vi "Write scan data array.vi"(8 "error in (no error)":errorcluster, 10 "scan data array":T1, 11 "Analysis in":refnum<class "Analysis.lvclass">) -> (0 "error out":errorcluster, 3 "Analysis out":refnum<class "Analysis.lvclass">)   [LabVIEW 2017, in "Analysis.lvclass"]
uses:
  Analysis.lvclass
  ScanDataArray_new.ctl
  Analysis.lvclass/Analysis.ctl
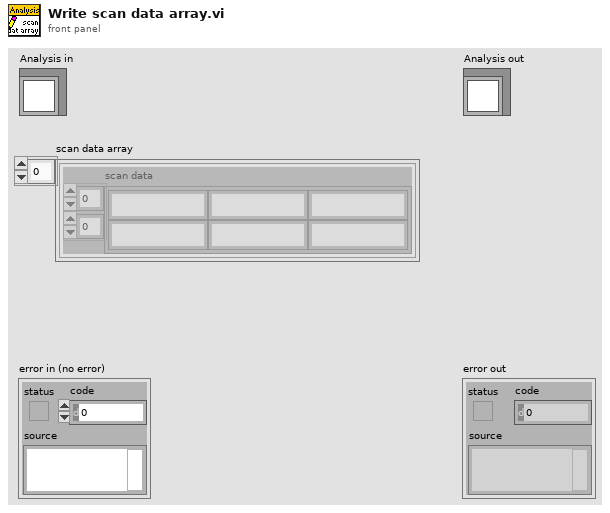
[diagram p1: front panel]
types:
  T1 = typedef "ScanDataArray_new.ctl" = cluster{"scan data":string[][]}[]
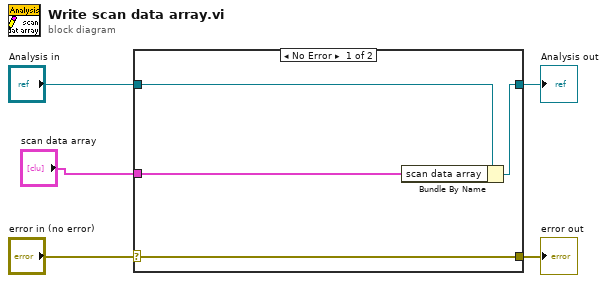
[diagram p0: block diagram]
diagram:
  n1 = case shown="No Error" "error in (no error)" {
    selector: "error in (no error)" -> [w9 w10]
    tunnel: [w9 w10] -> w4
    tunnel: [w7 w11] -> w2
    tunnel: "Analysis in" -> [w8 w11]
    tunnel: "scan data array" -> [w6 _]
    frame No Error {
      n2 = Bundle By Name(cluster=w8, "scan data array"=w6) -> (w7:refnum<class "Analysis.lvclass">)
    }
    frame Error {
    }
  }
  "error out" <- w4
  "Analysis out" <- w2
